vi "dsdll_capture_wave_get_status.vi"(8 "error in":errorcluster, 11 "dsdll instance in":T1={"dsdll path"=path "E:/LVprog/DirectSoundDLL/dsdll.dll", "dsdll handle"=[], "output devices"=[], "capture devices"=[]}) -> (0 "error out":errorcluster, 1 "progress [%]":i32, 2 "is capturing?":bool, 3 "dsdll instance out":T1, 4 "actual sample position":u32, 6 "total samples count":u32)   [LabVIEW 2013, in "dsdll.lvlib"]
doc: "Call this to get status of the recorder. Function can be anytime independetly to status of the recorder. It changes nothing in the DSDLL instance, so the 'dsdll instance out' is optional. Therefore it can be called from a different thread/process."
uses:
  dsdll.lvlib
  dsdll_instance.ctl
  dsdll_device_record.ctl
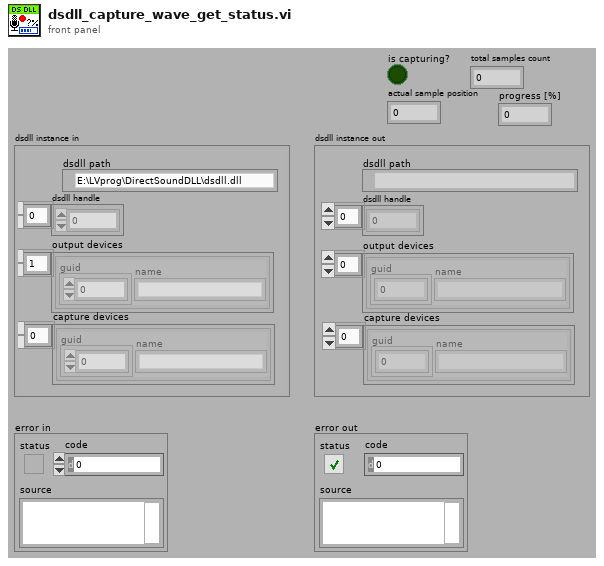
[diagram p1: front panel]
types:
  T1 = typedef "dsdll.lvlib/dsdll_instance.ctl" = cluster{"dsdll path":path, "dsdll handle":u8[], "output devices":T2[], "capture devices":T2[]}
  T2 = typedef "dsdll.lvlib/dsdll_device_record.ctl" = cluster{"guid":u8[], "name":string}
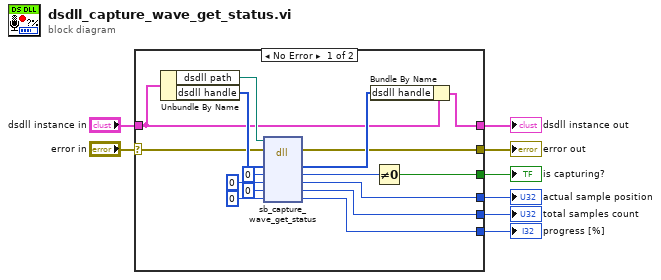
[diagram p0: block diagram]
diagram:
  n1 = case shown="No Error" "error in" {
    selector: "error in" -> [w9 w25]
    tunnel: [w21 w26] -> w8
    tunnel: [w15 _] -> w7
    tunnel: [w14 _] -> w6
    tunnel: [w13 _] -> w5
    tunnel: [w12 _] -> w4
    tunnel: [w11 w25] -> w3
    tunnel: "dsdll instance in" -> [w10 w26]
    frame No Error {
      n2 = Unbundle By Name(w10) -> ("dsdll path"=w23:path, "dsdll handle"=w22:u8[])
      n3 = dll-call lib="dsdll.dll" fn="sb_capture_wave_get_status" ("sb_get_handle_size()")(path in=w23, error in=w9, "handle"=w22, "status"=0, "smpl_pos"=u32 0, "smpl_count"=u32 0, "proc"=0) -> (error out=w11:errorcluster, "handle"=w24:u8[], "status"=w16:i32, "smpl_pos"=w14:u32, "smpl_count"=w13:u32, "proc"=w12:i32)  [unwired: 2 in, 1 out]
      n4 = Bundle By Name(cluster=w10, "dsdll handle"=w24) -> (w21:T1)
      n5 = Not Equal To 0?(x=w16) -> (x != 0?=w15:bool)
    }
    frame Error {
    }
  }
  "error out" <- w3
  "dsdll instance out" <- w8
  "is capturing?" <- w7
  "actual sample position" <- w6
  "total samples count" <- w5
  "progress [%]" <- w4
